vi "ex_4_2.vi"() -> ()   [LabVIEW 2020]
panel:
  out "Array 2":string[](array[string])
  in  "String":string
  out "Array":string[](array[string])
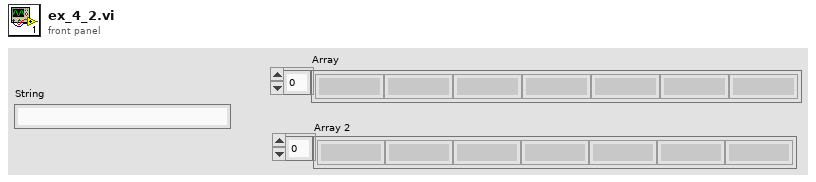
[diagram p1: front panel]
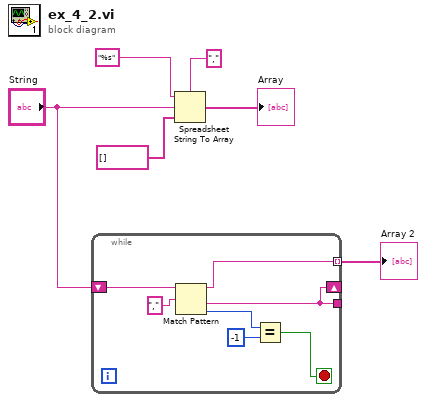
[diagram p0: block diagram]
diagram:
  n1 = while {
    shift-right: [w10] -> _
    shift-left: "String" -> [w13]
    tunnel: [w11] -> w1 mode=indexing
    tunnel: [w10] -> _
    stop <- w7 stop-if-true
    n2 = Match Pattern(string=w13, regular expression="," ("delimiter (Tab)")) -> (before substring=w11:string, after substring=w10:string, offset past match=w9:i32)  [unwired: 1 in, 1 out]
    n3 = Equal?(x=w9, y=-1) -> (x = y?=w7:bool)
  }
  "Array 2" <- w1
  n4 = Spreadsheet String To Array(delimiter (Tab)=",", format string="%s", spreadsheet string="String", array type (2D Dbl)=string[] []) -> (array=→"Array":string[])
